vi "Run FPGA Target VI.vi"(6 "clone#":i32, 8 "doneRef":refnum<vi>, 11 "targetVIref":T1) -> ()   [LabVIEW 2020, in "NI_TargetHelper.lvlib"]
uses:
  <vilib>/TargetSupport/NI_TargetHelper/NI_TargetHelper.lvlib
  <vilib>/TargetSupport/NI_TargetHelper/Instance VIref.ctl
  3e1c02f8-7f4a-2247-b090-43ad0878a07c.vi
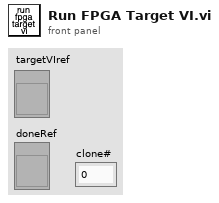
[diagram p1: front panel]
types:
  T1 = typedef "NI_TargetHelper.lvlib/Instance VIref.ctl" = refnum<vi>
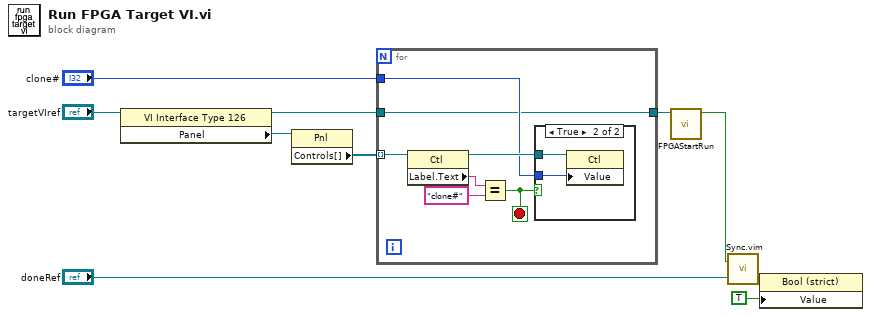
[diagram p0: block diagram]
diagram:
  n1 = property class="VI Interface Type 126"(reference="targetVIref") -> (reference out=w10:T1, "Panel"=w8:refnum<vi>)  [unwired: 1 in, 1 out]
  n2 = property class="Pnl"(reference=w8) -> ("Controls[]"=w9:refnum<vi>[])  [unwired: 1 in, 2 out]
  n3 = for {
    tunnel: w9 -> [w17] mode=indexing
    tunnel: "clone#" -> [w12]
    tunnel: [w11] -> w2
    tunnel: w10 -> [w11]
    stop <- w14 stop-if-true
    n4 = property class="Ctl"(reference=w17) -> (reference out=w13:refnum<vi>, "Label.Text"=w16:string)  [unwired: 1 in, 1 out]
    n5 = Equal?(x=w16, y="clone#") -> (x = y?=w14:bool)
    n6 = case shown="True" w14 {
      tunnel: w13 -> [_ w19]
      tunnel: w12 -> [_ w18]
      frame False {
      }
      frame True {
        n7 = property class="Ctl"(reference=w19, "Value"=w18) -> ()  [unwired: 1 in, 2 out]
      }
    }
  }
  n8 = call <vilib>:"FPGAStartRun.vi"("targetVIref"=w2) -> ("done"=w1:bool)  [unwired: 10 in]
  n9 = call "Sync.vim"("a"=w1, "b"="doneRef") -> ("b'"=w7:refnum<vi>)  [unwired: 24 in, 1 out]
  n10 = property class="Bool (strict)"(reference=w7, "Value"=TRUE) -> ()  [unwired: 1 in, 2 out]
